vi "ITX to LV 2.1 1D Variable Array Size.vi"(0 "file (use dialog)":path=path "P:/sample/GaAs/GaAs quantum dots/2008/PL Map/A1 735/060731ASBA_A1_6.0.itx") -> (2 "Array of clusters of wave data":cluster{"wave data":dbl[]}[](array[cluster]), 4 "wave names":string[](array[string]), 5 "Notes":string)   [LabVIEW 2016]
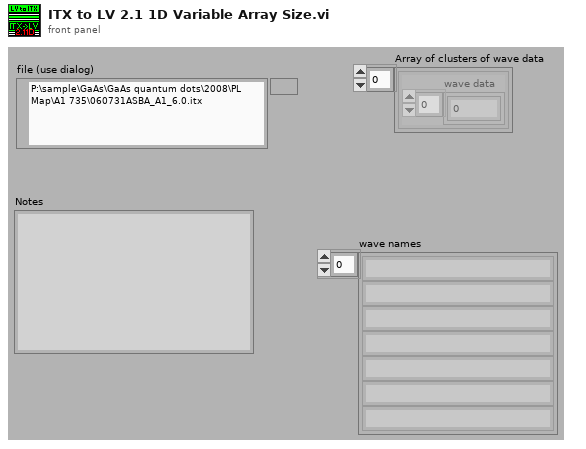
[diagram p1: front panel]
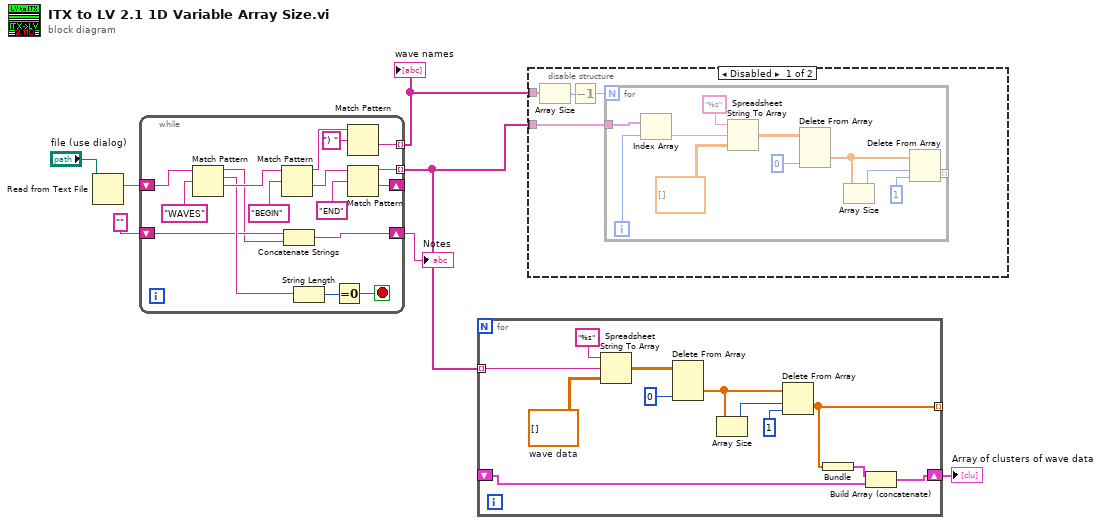
[diagram p0: block diagram]
diagram:
  n1 = Read from Text File(file (use dialog)="file (use dialog)") -> (text=w7:string)  [unwired: 2 in, 4 out]
  n2 = while {
    tunnel: [w8] -> w2 mode=indexing
    shift-right: [w22] -> _
    shift-left: w7 -> [w10]
    tunnel: [w18] -> w4 mode=indexing
    shift-right: [w13] -> w5
    shift-left: "" ("regular expression") -> [w12]
    stop <- w19 stop-if-true
    n3 = Match Pattern(string=w10, regular expression="WAVES") -> (before substring=w11:string, match substring=w21:string, after substring=w24:string)  [unwired: 2 out]
    n4 = Match Pattern(string=w24, regular expression="BEGIN" ("regular expression 2")) -> (before substring=w9:string, after substring=w23:string)  [unwired: 3 out]
    n5 = Concatenate Strings(w12, w11) -> (w13:string)
    n6 = String Length(string=w21) -> (length=w20:i32)
    n7 = Equal To 0?(x=w20) -> (x = 0?=w19:bool)
    n8 = Match Pattern(string=w9, regular expression=") ") -> (after substring=w18:string)  [unwired: 4 out]
    n9 = Match Pattern(string=w23, regular expression="END" ("regular expression 3")) -> (before substring=w8:string, after substring=w22:string)  [unwired: 3 out]
  }
  "wave names" <- w4
  "Notes" <- w5
  n10 = for {
    tunnel: [w28] -> _ mode=indexing
    tunnel: w2 -> [w29] mode=indexing
    shift-right: [w26] -> w1
    shift-left: _ -> [w25]
    w30 = dbl[][] []  # wave data
    n11 = Spreadsheet String To Array(format string="%s", spreadsheet string=w29, array type (2D Dbl)=w30) -> (array=w35:dbl[][])  [unwired: 1 out]
    n12 = Delete From Array(array=w35, index (col)=0 ("disabled index (col)")) -> (deleted portion=w34:dbl[])  [unwired: 2 in, 1 out]
    n13 = Array Size(array=w34) -> (size(s)=w33:i32)
    n14 = Delete From Array(array=w34, length=w33, index=1) -> (deleted portion=w28:dbl[])  [unwired: 1 out]
    n15 = Bundle("wave data"=w28) -> (w27:cluster{"wave data":dbl[]})  [unwired: 1 in]
    n16 = Build Array (concatenate)(w27, w25) -> (w26:cluster{"wave data":dbl[]}[])
  }
  "Array of clusters of wave data" <- w1
  n17 = disable-structure shown="Disabled" {
    disable-tunnel: w2 -> [w40 _]
    disable-tunnel: w4 -> [w39 _]
    frame Disabled {
      n18 = Array Size(array=w39) -> (size(s)=w38:i32)
      n19 = Decrement(x=w38) -> (x-1=w37:i32)
      n20 = for {
        N: w37 -> [_]
        tunnel: [w49] -> _ mode=indexing
        tunnel: w40 -> [w45]
        i -> [w41]
        n21 = Index Array(array=w45, index=w41) -> (element=w44:string)
        n22 = Spreadsheet String To Array(format string="%s", spreadsheet string=w44, array type (2D Dbl)=dbl[][] []) -> (array=w50:dbl[][])  [unwired: 1 out]
        n23 = Delete From Array(array=w50, index (col)=0 ("disabled index (col)")) -> (deleted portion=w48:dbl[])  [unwired: 2 in, 1 out]
        n24 = Array Size(array=w48) -> (size(s)=w47:i32)
        n25 = Delete From Array(array=w48, length=w47, index=1) -> (deleted portion=w49:dbl[])  [unwired: 1 out]
      }
    }
    frame Enabled {
    }
  }
